vi "Cube Logic Delayed Solinoid Status.vi"(8 "Short Input":bool, 11 "Long Input":bool) -> (0 "Short Delayed Output":bool, 3 "Long Delayed Output":bool)   [LabVIEW 2017]
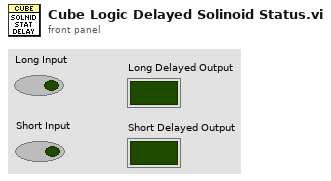
[diagram p1: front panel]
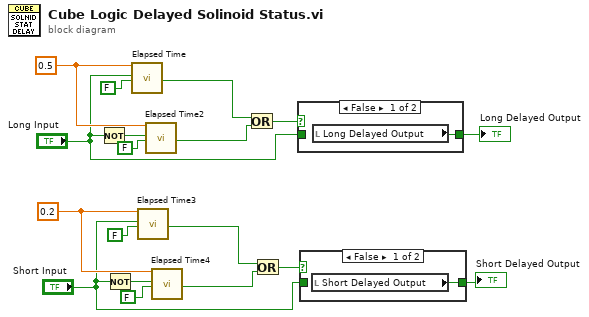
[diagram p0: block diagram]
diagram:
  w11 = 0.2 ("Time Target (s)")
  w12 = 0.5 ("Time Target (s)")
  n1 = Not(x="Long Input") -> (.not. x?=w18:bool)
  n2 = Not(x="Short Input") -> (.not. x?=w15:bool)
  n3 = call "Elapsed Time"("Time Target (s)"=w12, "Reset"="Long Input", "Auto Reset"=FALSE) -> ("Time has Elapsed"=w17:bool)  [unwired: 9 in, 7 out]
  n4 = call "Elapsed Time3"("Time Target (s)"=w11, "Reset"="Short Input", "Auto Reset"=FALSE) -> ("Time has Elapsed"=w14:bool)  [unwired: 9 in, 7 out]
  n5 = call "Elapsed Time2"("Time Target (s)"=w12, "Reset"=w18, "Auto Reset"=FALSE) -> ("Time has Elapsed"=w16:bool)  [unwired: 9 in, 7 out]
  n6 = call "Elapsed Time4"("Time Target (s)"=w11, "Reset"=w15, "Auto Reset"=FALSE) -> ("Time has Elapsed"=w13:bool)  [unwired: 9 in, 7 out]
  n7 = Or(x=w17, y=w16) -> (x .or. y?=w9:bool)
  n8 = Or(x=w14, y=w13) -> (x .or. y?=w10:bool)
  n9 = case shown="False" w9 {
    tunnel: "Long Input" -> [_ w20]
    tunnel: [w19 w20] -> w7
    frame False {
      n10 = local read "Long Delayed Output"() -> (w19:bool)
    }
    frame True {
    }
  }
  "Long Delayed Output" <- w7
  n11 = case shown="False" w10 {
    tunnel: "Short Input" -> [_ w22]
    tunnel: [w21 w22] -> w5
    frame False {
      n12 = local read "Short Delayed Output"() -> (w21:bool)
    }
    frame True {
    }
  }
  "Short Delayed Output" <- w5
